vi "v0.2_config_serial.vi"(4 "baud rate (9600/115200)":u32=9600, 5 "VISA COM IN":refnum<visa-resource-name>) -> (0 "error out":errorcluster, 2 "VISA COM OUT":refnum<visa-resource-name>)   [LabVIEW 2011]
doc: "<B>Configuración Serial</B>\n\nConecta mbed al PC mediante un puerto serial, dos velocidades son posibles: 9600/115200 baudios. Estas velocidades se setean desde el switch de configuración de la placa base."
uses:
  <vilib>/Instr/_visa.llb/VISA Configure Serial Port (Instr).vi
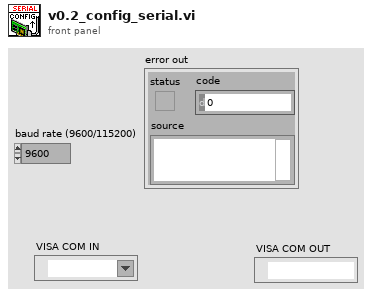
[diagram p1: front panel]
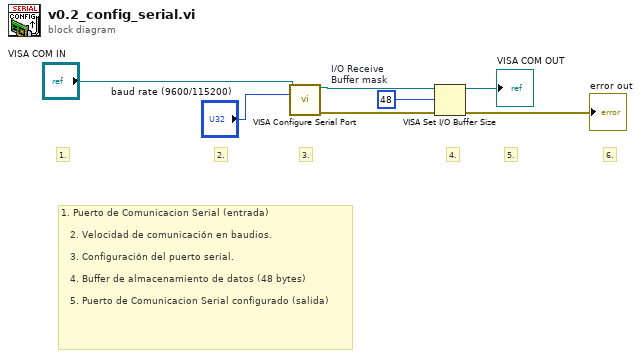
[diagram p0: block diagram]
diagram:
  w5 = u16 48  # I/O Receive Buffer mask
  # "1. Puerto de Comunicacion Serial (entrada)              \n\n   2. Velocidad de comunicación en baudios.\n\n   3. Configuración del puerto serial.\n\n   4. Buffer de almacenamiento de datos (48 bytes)\n\n   5. Puerto de Comunicacion Serial configurado (salida)"
  # "6."
  # "5."
  # "4."
  # "3."
  # "2."
  # "1."
  n1 = call-poly "VISA Configure Serial Port"("VISA resource name"="VISA COM IN", "baud rate (9600)"="baud rate (9600/115200)") -> ("VISA resource name out"=w6:refnum<visa-resource-name>, "error out"=w4:errorcluster)  [unwired: 12 in]
  n2 = VISA Set I/O Buffer Size(VISA resource name=w6, mask (16)=w5, error in (no error)=w4) -> (VISA resource name out=→"VISA COM OUT":refnum<visa-resource-name>, error out=→"error out":errorcluster)  [unwired: 1 in]
